vi "MouseOver.vi"(0 "reference in":refnum<class "Pgui_Obj.lvclass">, 1 "point":cluster{"x":i16, "y":i16}, 5 "error in (no error)":errorcluster) -> (14 "reference out":refnum<class "Pgui_Obj.lvclass">, 19 "error out":errorcluster)   [LabVIEW 2019, in "Pgui_Obj.lvclass"]
uses:
  Pgui_Obj.lvclass
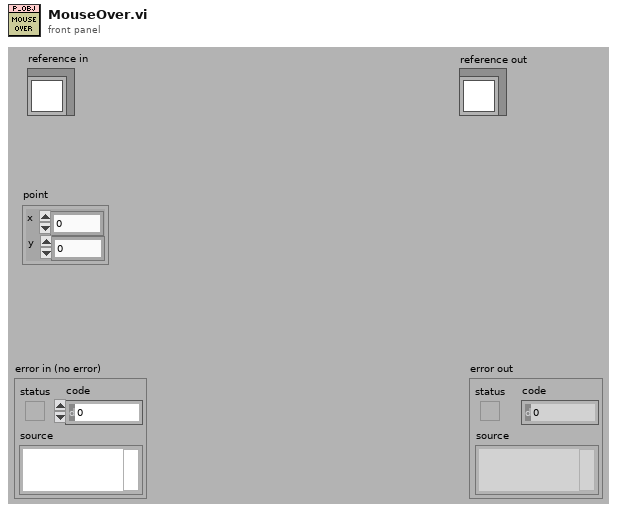
[diagram p1: front panel]
types:
  T1 = cluster{"left":i16, "top":i16, "right":i16, "bottom":i16}
  T2 = typedef "Pgui_Obj.lvclass/ObjectAttributes.ctl" = cluster{"Children":refnum<class "Pgui_Obj.lvclass">[], "Draw Instr":picture, "Params":cluster{"left":i16, "top":i16, "right":i16, "bottom":i16}, "Parent_Pgui_Obj":refnum<class "Pgui_Obj.lvclass">, "MouseOver":bool}
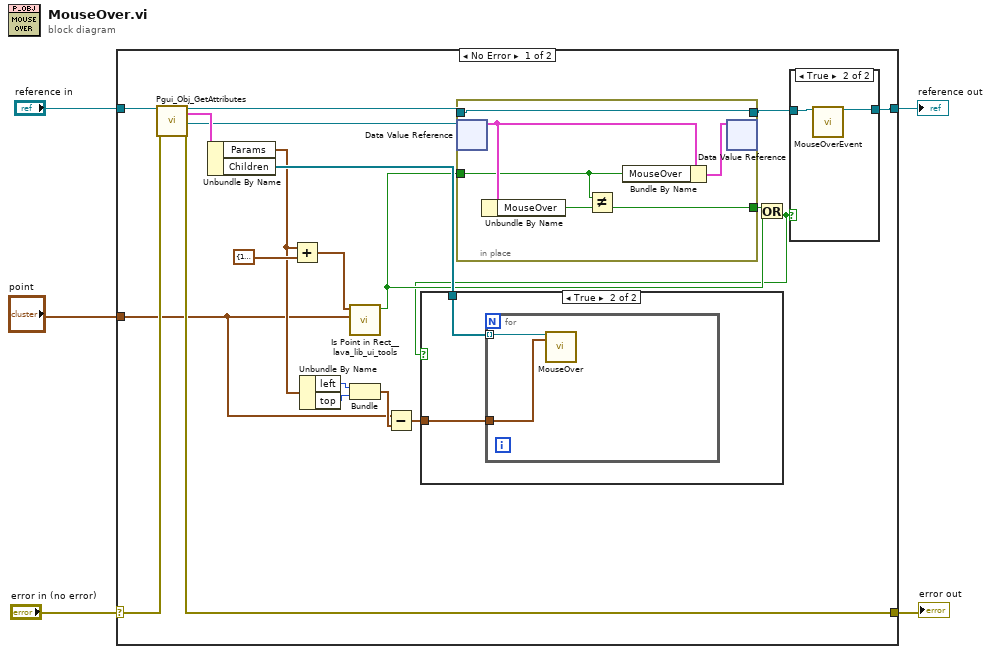
[diagram p0: block diagram]
diagram:
  n1 = case shown="No Error" "error in (no error)" {
    selector: "error in (no error)" -> [w25 w40]
    tunnel: [w23 w40] -> w4
    tunnel: [w10 w39] -> w2
    tunnel: "reference in" -> [w22 w39]
    tunnel: "point" -> [w6 _]
    frame No Error {
      n2 = call "Pgui_Obj_GetAttributes.vi"("reference in"=w22, "error in (no error)"=w25) -> ("reference out"=w11:refnum<class "Pgui_Obj.lvclass">, "Data"=w24:T2, "DataRef"=w19:refnum<data-value>, "error out"=w23:errorcluster)  [unwired: 14 in]
      n3 = Unbundle By Name(w24) -> ("Params"=w14:T1, "Children"=w18:refnum<class "Pgui_Obj.lvclass">[])
      n4 = Add(x=w14, y=T1 {"left"=1, "top"=1, "right"=-1, "bottom"=-1} ("Params")) -> (x+y=w20:T1)
      n5 = Unbundle By Name(w14) -> ("left"=w15:i16, "top"=w16:i16)
      n6 = call <vilib>:"Is Point in Rect__lava_lib_ui_tools.vi"("point"=w6, "rect"=w20) -> ("Point in Rect?"=w13:bool)  [unwired: 9 in]
      n7 = Bundle("left"=w15, "top"=w16) -> (w17:cluster{"left":i16, "top":i16})  [unwired: 1 in]
      n8 = Subtract(x=w6, y=w17) -> (x-y=w7:cluster{i16, i16})
      n9 = in-place {
        in-place-border: w13 -> [w34]
        in-place-border: [w37] -> w12
        in-place-border: w11 -> [w37]
        in-place-border: [w33] -> w9
        n10 = in-place-dvr #1(w19) -> (w36:T2)  [unwired: 1 out]
        n11 = Unbundle By Name(w36) -> ("MouseOver"=w35:bool)
        n12 = Not Equal?(x=w34, y=w35) -> (x != y?=w33:bool)
        n13 = Bundle By Name(cluster=w36, "MouseOver"=w34) -> (w38:T2)
        n14 = in-place-dvr #1(w38) -> ()  [unwired: 2 out]
      }
      n15 = Or(x=w9, y=w13) -> (x .or. y?=w8:bool)
      n16 = case shown="True" w8 {
        tunnel: w18 -> [_ w30]
        tunnel: w7 -> [_ w29]
        frame False {
        }
        frame True {
          n17 = for {
            tunnel: w30 -> [w32] mode=indexing
            tunnel: w29 -> [w31]
            n18 = call-dynamic "MouseOver.vi"("reference in"=w32, "point"=w31) -> ()  [unwired: 16 in, 2 out]
          }
        }
      }
      n19 = case shown="True" w8 {
        tunnel: w12 -> [w26 w28]
        tunnel: [w26 w27] -> w10
        frame False {
        }
        frame True {
          n20 = call-dynamic "MouseOverEvent.vi"("reference in"=w28) -> ("reference out"=w27:refnum<class "Pgui_Obj.lvclass">)  [unwired: 17 in, 1 out]
        }
      }
    }
    frame Error {
    }
  }
  "error out" <- w4
  "reference out" <- w2
